vi "Check Dilate Changed.vi"(11 "Dilate":refnum<vi>) -> ()   [LabVIEW 2025]
uses:
  <vilib>/Rock Robotics/Network Tables/NT Read Boolean.vi
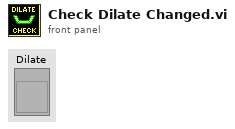
[diagram p1: front panel]
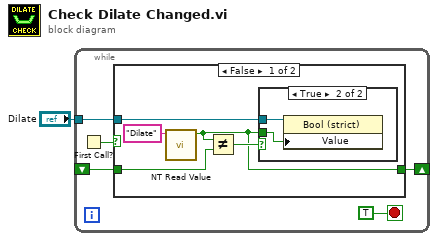
[diagram p0: block diagram]
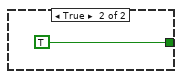
[diagram p3: hidden frame]
diagram:
  n1 = while {
    shift-right: [w5] -> _
    shift-left: _ -> [w4]
    tunnel: "Dilate" -> [w2]
    stop <- TRUE stop-if-true
    n2 = First Call?() -> (First Call?: T/F=w6:bool)
    n3 = case shown="False" w6 {
      tunnel: [w7 TRUE] -> w5
      tunnel: w4 -> [w11 _]
      tunnel: w2 -> [w8 _]
      frame False {
        n4 = call-poly <vilib>:"NT Read Value.vi"("name"="Dilate" ("Name")) -> ("value"=w7:bool)  [unwired: 8 in, 2 out]
        n5 = Not Equal?(x=w7, y=w11) -> (x != y?=w9:bool)
        n6 = case shown="True" w9 {
          tunnel: w8 -> [_ w13]
          tunnel: w7 -> [_ w12]
          frame False {
          }
          frame True {
            n7 = property class="Bool (strict)"(reference=w13, "Value"=w12) -> ()  [unwired: 1 in, 2 out]
          }
        }
      }
      frame True {
      }
    }
  }
